vi "Wait For Signal Bank.vi"(8 "error in (no error)":errorcluster, 10 "timeout (ms)":i32=5000) -> (0 "error out":errorcluster={"status"=TRUE, "code"=555, "source"="Timed out waiting for Signal Bank."}, 2 "PauseDAQ":bool)   [LabVIEW 2020]
uses:
  PXI Globals.vi
panel:
  out "Elapsed time (ms)":u32
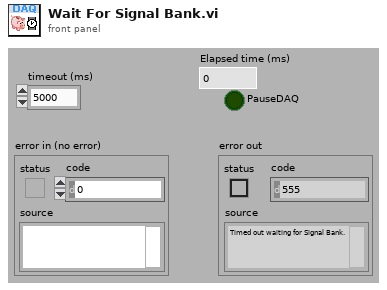
[diagram p1: front panel]
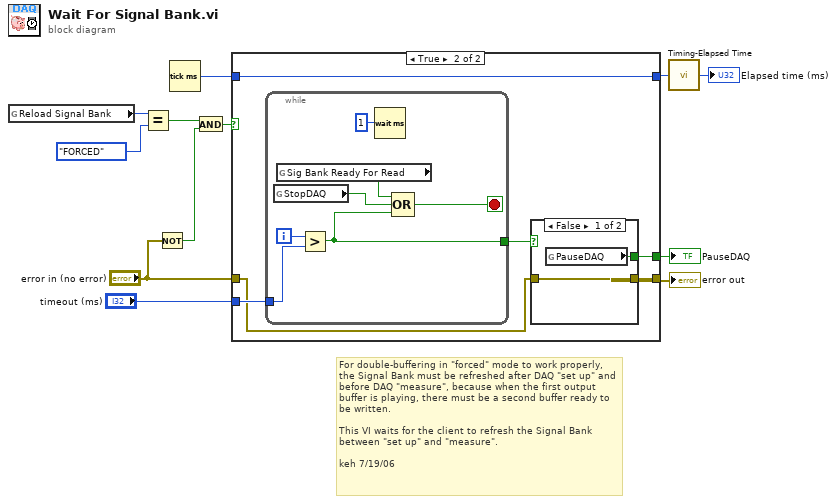
[diagram p0: block diagram]
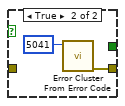
[diagram p3: hidden frame]
diagram:
  # "For double-buffering in \"forced\" mode to work properly, the Signal Bank must be refreshed after DAQ \"set up\" and before DAQ \"measure\", because when the first output buffer is playing, there must be a second buffer ready to be written. \n\nThis VI waits for the client to refresh the Signal Bank between \"set up\" and \"measure\".\n\nkeh 7/19/06"
  n1 = global read "PXI Globals.vi" "Reload Signal Bank"() -> (w12:enum32{"OFF", "ENABLED", "FORCED"})
  n2 = Equal?(x=w12, y=enum16{"OFF", "ENABLED", "FORCED"}."FORCED") -> (x = y?=w6:bool)
  n3 = Not(x="error in (no error)") -> (.not. x?=w9:bool)
  n4 = Tick Count (ms)() -> (millisecond timer value=w3:u32)
  n5 = And(x=w6, y=w9) -> (x .and. y?=w8:bool)
  n6 = case shown="True" w8 {
    tunnel: "error in (no error)" -> [w13 w16]
    tunnel: [w13 w18] -> w10
    tunnel: "timeout (ms)" -> [_ w17]
    tunnel: [_ w15] -> w5
    tunnel: w3 -> [_ w14]
    tunnel: [_ w14] -> w2
    frame False {
    }
    frame True {
      n7 = while {
        tunnel: w17 -> [w27]
        tunnel: [w25] -> w19
        i -> [w28]
        stop <- w30 stop-if-true
        n8 = global read "PXI Globals.vi" "StopDAQ"() -> (w26:bool)
        n9 = global read "PXI Globals.vi" "Sig Bank Ready For Read"() -> (w29:bool)
        n10 = Greater?(x=w28, y=w27) -> (0:w25:bool)
        n11 = Wait (ms)(milliseconds to wait=1) -> ()  [unwired: 1 out]
        n12 = Compound Arithmetic op=OR(w29, w26, w25) -> (w30:bool)
      }
      n13 = case shown="False" w19 {
        tunnel: w16 -> [w21 _]
        tunnel: [w21 w23] -> w18
        tunnel: [w20 _] -> w15
        frame False {
          n14 = global read "PXI Globals.vi" "PauseDAQ"() -> (w20:bool)
        }
        frame True {
          n15 = call <vilib>:"Error Cluster From Error Code.vi"("error code (0)"=5041) -> ("error out"=w23:errorcluster)  [unwired: 8 in]
        }
      }
    }
  }
  "error out" <- w10
  "PauseDAQ" <- w5
  n16 = call "Timing-Elapsed Time.vi"("Start time (ms)"=w2) -> ("Elapsed time (ms)"=→"Elapsed time (ms)":u32)  [unwired: 4 in]
